vi "FTW-TestExecutive-Core_Abort.vi"(0 "FTW-TestExecutive-Core In":refnum<class "FTW-TestExecutive-Core.lvclass">, 11 "error in":errorcluster) -> (4 "FTW-TestExecutive-Core Out":refnum<class "FTW-TestExecutive-Core.lvclass">, 15 "error out":errorcluster)   [LabVIEW 2015, in "FTW-TestExecutive-Core.lvclass"]
uses:
  FTW-TestExecutive-Core.lvclass
  FTW-TestExecutive-Core.lvclass/FTW-TestExecutive-Core.ctl
  FTW-TestExecutive-Step-State.ctl
  FTW-TestExecutive-Core_State.ctl
  Connector/FTW-ActorConnector.lvclass
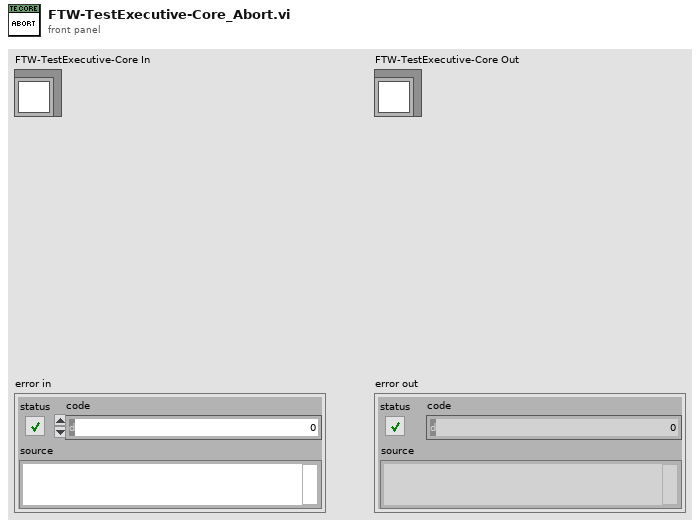
[diagram p1: front panel]
types:
  T1 = typedef "FTW-TestExecutive-Core.lvclass/FTW-TestExecutive-Core_State.ctl" = enum8{"Unloaded", "Loaded", "Executing", "Paused"}
  T2 = typedef "FTW-TestExecutive-Step-State.ctl" = enum8{"None", "Failed", "Passed", "Timed out", "Aborted"}
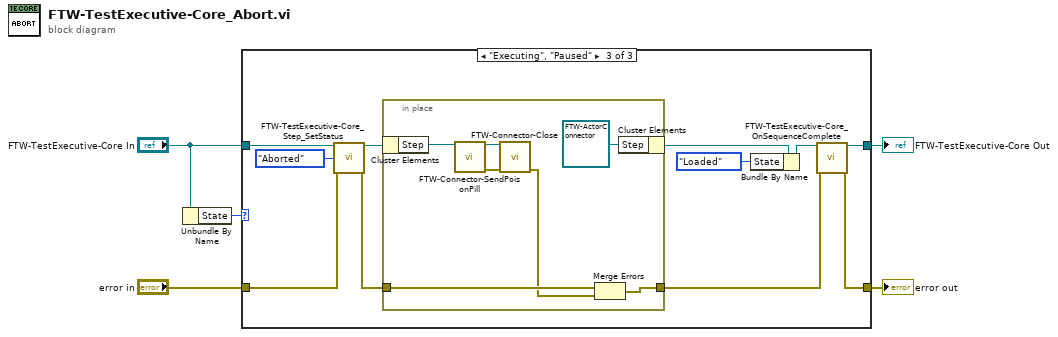
[diagram p0: block diagram]
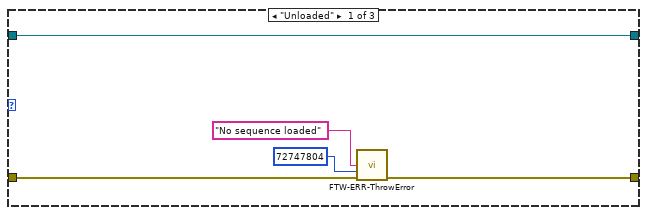
[diagram p2: hidden frame]
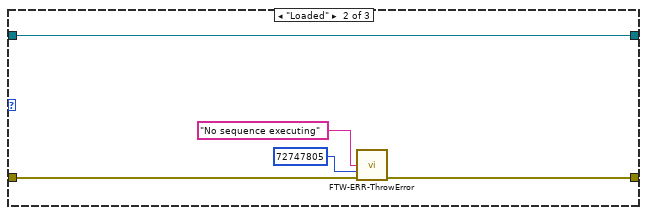
[diagram p3: hidden frame]
diagram:
  n1 = Unbundle By Name("FTW-TestExecutive-Core In") -> ("State"=w3:T1)
  n2 = case shown="\"Executing\", \"Paused\"" w3 {
    tunnel: [w10 w15 w21] -> w5
    tunnel: "FTW-TestExecutive-Core In" -> [w10 w15 w26]
    tunnel: [w8 w13 w20] -> w2
    tunnel: "error in" -> [w9 w14 w24]
    frame "Unloaded" {
      n3 = call "FTW-ERR-ThrowError.vi"("Error Message"="No sequence loaded", "Error Code"=72747804, "error in"=w9) -> ("error out"=w8:errorcluster)  [unwired: 12 in]
    }
    frame "Loaded" {
      n4 = call "FTW-ERR-ThrowError.vi"("Error Message"="No sequence executing", "Error Code"=72747805, "error in"=w14) -> ("error out"=w13:errorcluster)  [unwired: 12 in]
    }
    frame "Executing", "Paused" {
      n5 = call "FTW-TestExecutive-Core_Step_SetStatus.vi"("FTW-TestExecutive-Core In"=w26, "State"=FTW-TestExecutive-Step-State."Aborted", "error in"=w24) -> ("FTW-TestExecutive-Core Out"=w17:refnum<class "FTW-TestExecutive-Core.lvclass">, "error out"=w18:errorcluster)  [unwired: 11 in]
      n6 = in-place {
        in-place-border: [w28] -> w19
        in-place-border: w18 -> [w33]
        n7 = in-place-cluster #1(w17) -> ("Step"=w29:refnum<class "FTW-ActorConnector.lvclass">)
        n8 = call-dynamic "FTW-Connector-SendPoisonPill.vi"("FTW Actor Connector"=w29) -> ("FTW Actor Connector out"=w31:refnum<class "FTW-ActorConnector.lvclass">, "error out"=w30:errorcluster)  [unwired: 9 in, 4 out]
        n9 = call-dynamic "FTW-Connector-Close.vi"("FTW Actor Connector"=w31, "error in"=w30) -> ("error out"=w27:errorcluster)  [unwired: 13 in]
        n10 = Merge Errors(w33, w27) -> (w28:errorcluster)
        n11 = in-place-cluster #1("Step"=refnum<class "FTW-ActorConnector.lvclass"> refnum) -> (w16:refnum<class "FTW-TestExecutive-Core.lvclass">)
      }
      n12 = Bundle By Name(cluster=w16, "State"=FTW-TestExecutive-Core_State."Loaded") -> (w23:refnum<class "FTW-TestExecutive-Core.lvclass">)
      n13 = call "FTW-TestExecutive-Core_OnSequenceComplete.vi"("FTW-TestExecutive-Core In"=w23, "error in"=w19) -> ("FTW-TestExecutive-Core Out"=w21:refnum<class "FTW-TestExecutive-Core.lvclass">, "error out"=w20:errorcluster)  [unwired: 12 in]
    }
  }
  "FTW-TestExecutive-Core Out" <- w5
  "error out" <- w2
